vi "Speed Estimation.vi"   [LabVIEW 2016, in "NI_EP_Motor Monitoring.lvlib"]
doc: "Calculates the motor speed. You must manually select the polymorphic instance you want to use."
uses:
  <vilib>/addons/Electrical Power/Motor Monitoring/NI_EP_Motor Monitoring.lvlib
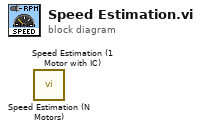
[diagram p0: block diagram]
diagram:
  n1 = call <vilib>:"Speed Estimation (N Motors).vi"() -> ()  [unwired: 12 in, 4 out]
  n2 = call <vilib>:"Speed Estimation (1 Motor with IC).vi"() -> ()  [unwired: 11 in, 5 out]
